vi "Start all VIs Globals.vi"() -> ()   [LabVIEW 2014]
panel:
  in  "VI Paths":T1={"Shutter Control"=path "C:/Users/Lambda2/Desktop/Testing/Testing-Lambda/Testing/Shutter Control", "Stage Control"=path "C:/Users/Lambda2/Desktop/Testing/Testing-Lambda/Testing/Stage Control", "Camera & Acquisition VIs"=path "C:/Users/Lambda2/Desktop/Testing/Testing-Lambda/Testing/Camera & acquisition VIs", "TIRF Lock"=path "C:/Users/Lambda2/Desktop/Testing/Testing-Lambda/Testing/TIRF Lock"}
  in  "VIs to Run":T2(array[cluster])=[{"VI Name"="shutter-control.vi", "Location"=enum."Shutter Control", "Run?"=TRUE, "Minimized?"=FALSE, "Subdirectory (w trailing \"/\")"="Shutter SubVIs\\"}, {"VI Name"="stage-controller.vi", "Location"=enum."Stage Control", "Run?"=TRUE, "Minimized?"=FALSE, "Subdirectory (w trailing \"/\")"="Stage SubVIs\\"}, {"VI Name"="camera-startup.vi", "Location"=enum."Camera & Acquisition VIs", "Run?"=TRUE, "Minimized?"=FALSE, "Subdirectory (w trailing \"/\")"="SubVIs\\"}, {"VI Name"="autofocus-globals.vi", "Location"=enum."TIRF Lock", "Run?"=TRUE, "Minimized?"=FALSE, "Subdirectory (w trailing \"/\")"=""}, {"VI Name"="autofocus-view-calibration.vi", "Location"=enum."TIRF Lock", "Run?"=TRUE, "Minimized?"=FALSE, "Subdirectory (w trailing \"/\")"="TIRF\\"}, {"VI Name"="multi-mode-acquisition.vi", "Location"=enum."Camera & Acquisition VIs", "Run?"=TRUE, "Minimized?"=FALSE, "Subdirectory (w trailing \"/\")"="SubVIs\\"}, {"VI Name"="Camera-SetUp-Acquisition.vi", "Location"=enum."Camera & Acquisition VIs", "Run?"=TRUE, "Minimized?"=FALSE, "Subdirectory (w trailing \"/\")"="SubVIs\\"}, {"VI Name"="z-stack acquistion.vi", "Location"=enum."Camera & Acquisition VIs", "Run?"=TRUE, "Minimized?"=TRUE, "Subdirectory (w trailing \"/\")"="SubVIs\\"}]
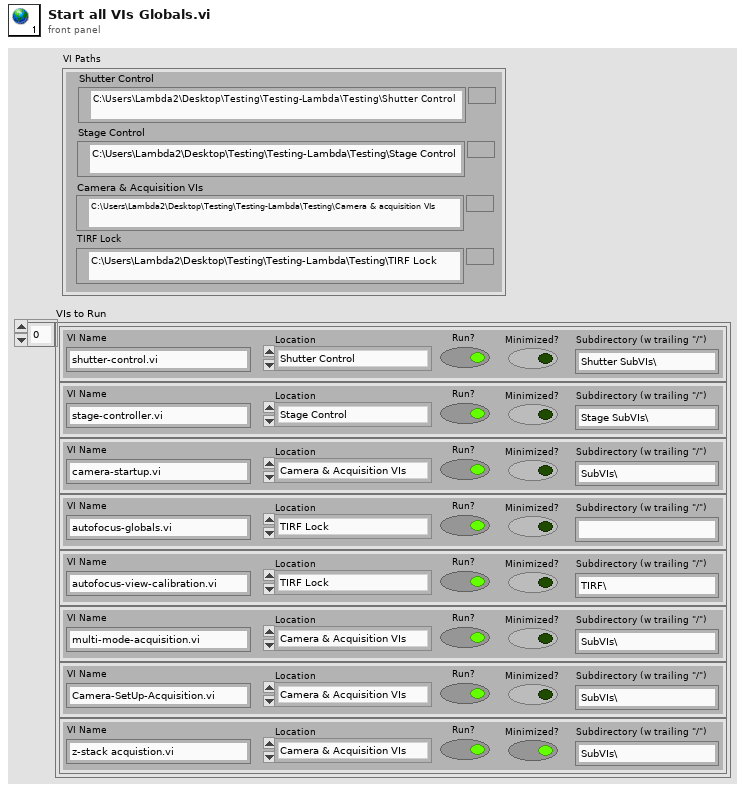
[diagram p1: front panel]
types:
  T1 = cluster{"Shutter Control":path, "Stage Control":path, "Camera & Acquisition VIs":path, "TIRF Lock":path}
  T2 = cluster{"VI Name":string, "Location":enum16{"TIRF Lock", "Camera & Acquisition VIs", "Stage Control", "Shutter Control"}, "Run?":bool, "Minimized?":bool, "Subdirectory (w trailing \"/\")":string}[]
diagram:
